vi "换算-秒至天以内.vi"(11 "秒":dbl=223.0 format="%#_13g") -> (0 "s":dbl, 1 "m":dbl, 2 "h":dbl, 3 "d":dbl)   [LabVIEW 2017]
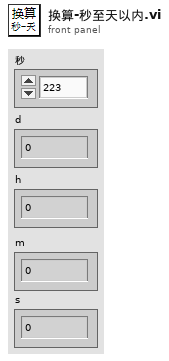
[diagram p1: front panel]
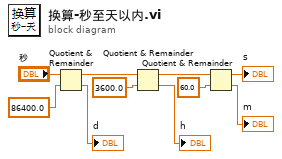
[diagram p0: block diagram]
diagram:
  n1 = Quotient & Remainder(x="秒", y=86400.0) -> (x-y*floor(x/y)=w6:dbl, floor(x/y)=→"d":dbl)
  n2 = Quotient & Remainder(x=w6, y=3600.0) -> (x-y*floor(x/y)=w5:dbl, floor(x/y)=→"h":dbl)
  n3 = Quotient & Remainder(x=w5, y=60.0) -> (x-y*floor(x/y)=→"s":dbl, floor(x/y)=→"m":dbl)
